vi "GetTestFile_testItem.vi"(11 "Program path":path) -> (2 "转置的数组":string[][](array[string]), 3 "路径输出":path)   [LabVIEW 2018]
uses:
  Global.vi
panel:
  out "error out":errorcluster caption="错误输出"
  in  "error in (no error)":errorcluster caption="错误输入（无错误）"
  out "数组 2":string[](array[string])
  out "数组":string[](array[string])
  out "文件名":string[](array[string])
  # "C:\\Users\\Administrator\\Desktop\\ATE_Program\\ModelInformation"
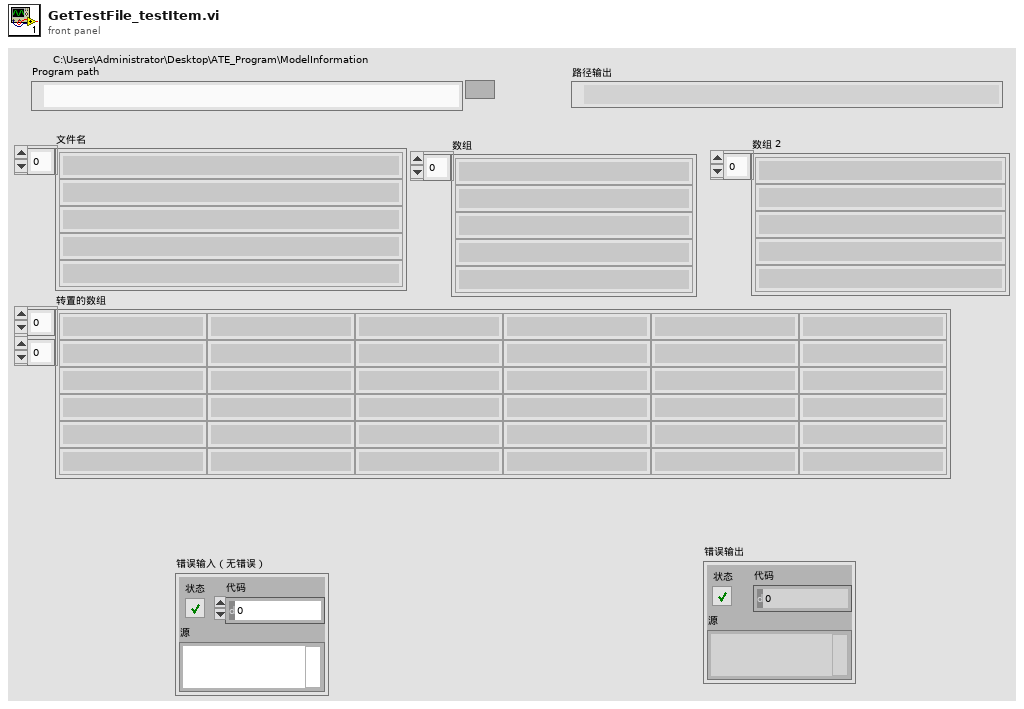
[diagram p1: front panel]
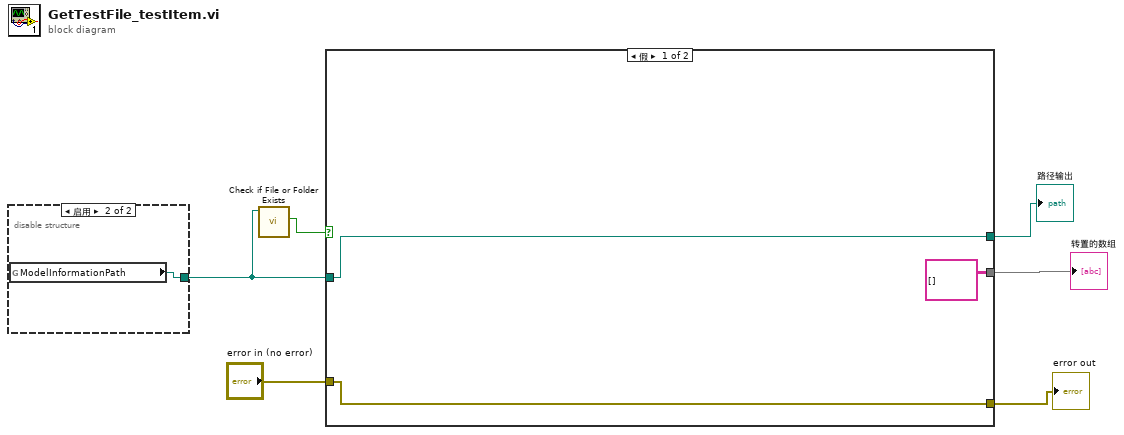
[diagram p0: block diagram]
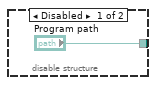
[diagram p2: hidden frame]
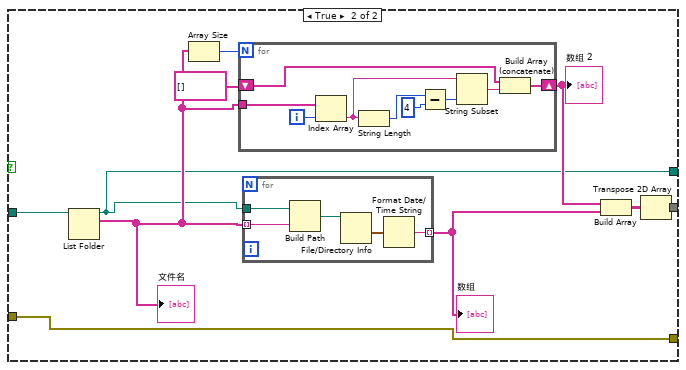
[diagram p3: hidden frame]
diagram:
  n1 = disable-structure shown="启用" {
    disable-tunnel: ["Program path" w8] -> w4
    frame Disabled {
    }
    frame Enabled {
      n2 = global read "Global.vi" "ModelInformationPath"() -> (w8:path)
    }
  }
  n3 = call <vilib>:"Check if File or Folder Exists.vi"("path"=w4) -> ("file or folder exists?"=w3:bool)  [unwired: 8 in, 2 out]
  n4 = case shown="假" w3 {
    tunnel: w4 -> [w11 w21]
    tunnel: [string[][] [] w14] -> w6
    tunnel: [w11 w13] -> w5
    tunnel: [w9 w12] -> w2
    tunnel: "error in (no error)" -> [w9 w12]
    frame False {
    }
    frame True {
      n5 = List Folder(path=w21) -> (path out=w13:path, filenames=w18:string[])  [unwired: 1 in, 4 out]
      "文件名" <- w18
      n6 = Array Size(array=w18) -> (size(s)=w19:i32)
      n7 = for {
        N: w19 -> [_]
        tunnel: w18 -> [w30]
        shift-right: [w23] -> w16
        shift-left: string[] [] -> [w22]
        i -> [w29]
        n8 = Index Array(array=w30, index=w29) -> (element=w26:string)
        n9 = String Length(string=w26) -> (length=w28:i32)
        n10 = Subtract(x=w28, y=4) -> (x-y=w25:i32)
        n11 = String Subset(string=w26, length (rest)=w25) -> (substring=w24:string)  [unwired: 1 out]
        n12 = Build Array (concatenate)(w22, w24) -> (w23:string[])
      }
      "数组 2" <- w16
      n13 = for {
        tunnel: w18 -> [w34] mode=indexing
        tunnel: w13 -> [w35]
        tunnel: [w31] -> w15 mode=indexing
        n14 = Build Path(base path=w35, name or relative path=w34) -> (appended path=w33:path)
        n15 = File/Directory Info(path=w33) -> (last mod=w32:timestamp)  [unwired: 1 in, 6 out]
        n16 = Format Date/Time String(seconds (now)=w32) -> (date/time string=w31:string)  [unwired: 2 out]
      }
      "数组" <- w15
      n17 = Build Array(w16, w15) -> (w17:string[][])
      n18 = Transpose 2D Array(2D array=w17) -> (transposed array=w14:string[][])
    }
  }
  "转置的数组" <- w6
  "路径输出" <- w5
  "error out" <- w2
